vi "Rearrange Functions.vi"(11 "Functions in":T1[](array[typedef])) -> (3 "Functions in":T1[](array[typedef]))   [LabVIEW 2021, in "TAF Proj Document Type.lvlib" / "Dqmh Module.lvclass"]
uses:
  <vilib>/Wovalab/AntiDoc/Document Type/Add-ons/LabVIEW TAF Project/Dqmh Module/Dqmh Module.lvclass
  <vilib>/Wovalab/AntiDoc/Document Type/Add-ons/LabVIEW TAF Project/Dqmh Module/Requests Used By Module--cluster.ctl
  <vilib>/Wovalab/AntiDoc/Document Type/Add-ons/LabVIEW TAF Project/Project Parser/Module Fonctions--cluster.ctl
  <vilib>/Wovalab/AntiDoc/Document Type/Add-ons/LabVIEW TAF Project/Project Parser/Project Parser.lvlib
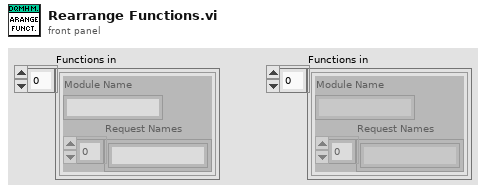
[diagram p1: front panel]
types:
  T1 = typedef "TAF Proj Document Type.lvlib/Dqmh Module.lvclass/Requests Used By Module--cluster.ctl" = cluster{"Module Name":string, "Request Names":string[]}
  T2 = typedef "TAF Proj Document Type.lvlib/Project Parser.lvlib/Module Fonctions--cluster.ctl" = cluster{"Module Name":string, "Functions":string[]}
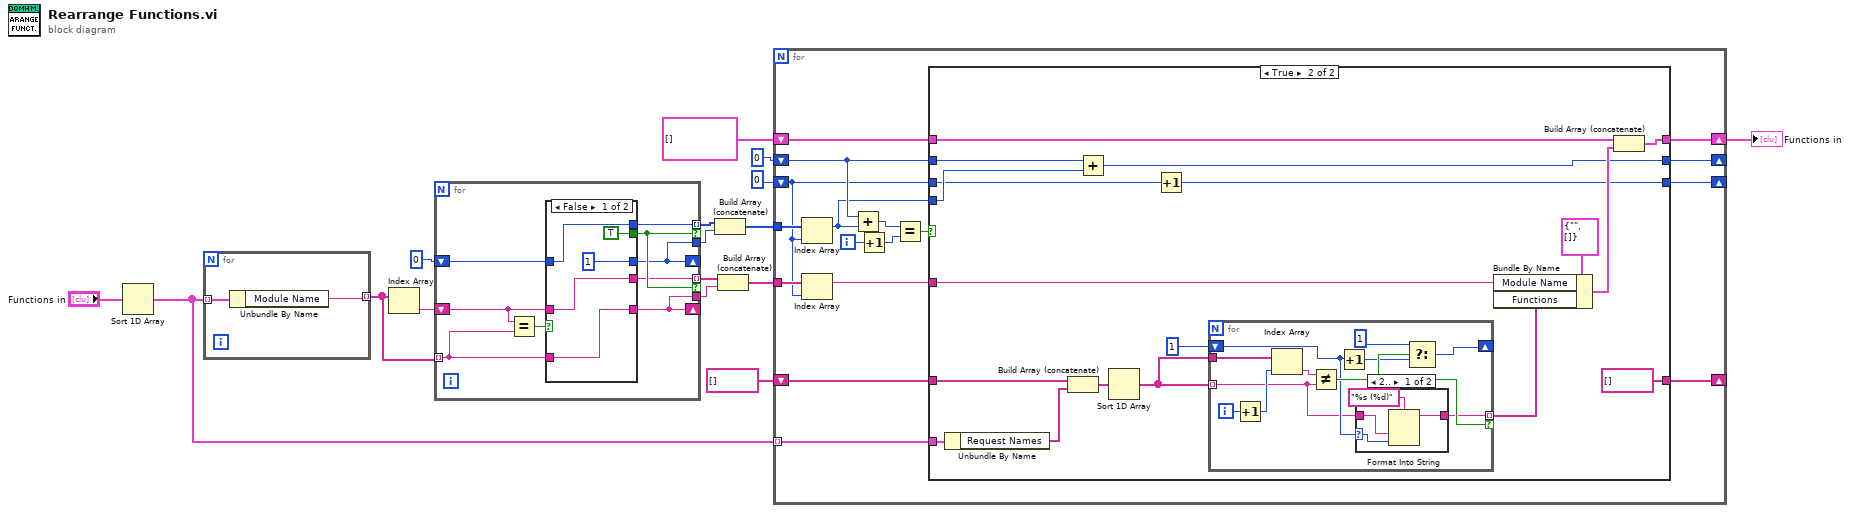
[diagram p0: block diagram]
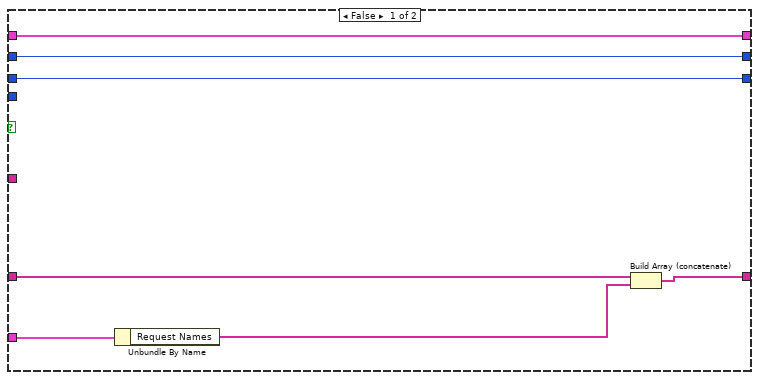
[diagram p2: hidden frame]
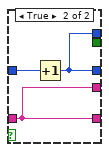
[diagram p4: hidden frame]
diagram:
  n1 = Sort 1D Array(array="Functions in") -> (sorted array=w1:T1[])
  n2 = for {
    tunnel: w1 -> [w18] mode=indexing
    tunnel: [w17] -> w11 mode=indexing
    n3 = Unbundle By Name(w18) -> ("Module Name"=w17:string)
  }
  n4 = Index Array(array=w11) -> (element=w10:string)  [unwired: 1 in]
  n5 = for {
    tunnel: w11 -> [w25] mode=indexing
    shift-right: [w19] -> _
    shift-left: w10 -> [w26]
    shift-right: [w20] -> _
    shift-left: 0 -> [w27]
    tunnel: [w22] -> w13 mode=indexing if=w24
    tunnel: [w21] -> w16 mode=indexing if=w24
    tunnel: [w20] -> w14
    tunnel: [w19] -> w15
    n6 = Equal?(x=w26, y=w25) -> (x = y?=w23:bool)
    n7 = case shown="False" w23 {
      tunnel: w27 -> [w32 w35]
      tunnel: [1 w33] -> w20
      tunnel: [w32 w33] -> w22
      tunnel: [w28 w34] -> w19
      tunnel: w25 -> [w28 _]
      tunnel: w26 -> [w29 w34]
      tunnel: [w29 w34] -> w21
      tunnel: [TRUE _] -> w24
      frame False {
      }
      frame True {
        n8 = Increment(x=w35) -> (x+1=w33:i32)
      }
    }
  }
  n9 = Build Array (concatenate)(w13, w14) -> (w6:i32[])
  n10 = Build Array (concatenate)(w16, w15) -> (w5:string[])
  n11 = for {
    tunnel: w1 -> [w36] mode=indexing
    tunnel: w5 -> [w47]
    tunnel: w6 -> [w51]
    shift-right: [w48] -> w9
    shift-left: T2[] [] ("Registred Broadcast") -> [w49]
    shift-right: [w45] -> _
    shift-left: string[] [] ("appended array") -> [w46]
    shift-right: [w43] -> _
    shift-left: 0 -> [w41]
    shift-right: [w38] -> _
    shift-left: 0 -> [w39]
    i -> [w52]
    n12 = Index Array(array=w51, index=w39) -> (element=w37:i32)
    n13 = Index Array(array=w47, index=w39) -> (element=w40:string)
    n14 = Add(x=w41, y=w37) -> (x+y=w42:i32)
    n15 = Increment(x=w52) -> (x+1=w44:i32)
    n16 = Equal?(x=w42, y=w44) -> (x = y?=w50:bool)
    n17 = case shown="True" w50 {
      tunnel: w49 -> [w59 w75]
      tunnel: [w59 w74] -> w48
      tunnel: w40 -> [_ w73]
      tunnel: w46 -> [w58 w65]
      tunnel: [w53 string[] []] -> w45
      tunnel: w37 -> [_ w72]
      tunnel: w41 -> [w57 w71]
      tunnel: [w57 w70] -> w43
      tunnel: w39 -> [w56 w69]
      tunnel: [w56 w68] -> w38
      tunnel: w36 -> [w55 w67]
      frame False {
        n18 = Unbundle By Name(w55) -> ("Request Names"=w54:string[])
        n19 = Build Array (concatenate)(w58, w54) -> (w53:string[])
      }
      frame True {
        n20 = Unbundle By Name(w67) -> ("Request Names"=w66:string[])
        n21 = Build Array (concatenate)(w65, w66) -> (w63:string[])
        n22 = Add(x=w71, y=w72) -> (x+y=w70:i32)
        n23 = Sort 1D Array(array=w63) -> (sorted array=w61:string[])
        n24 = Increment(x=w69) -> (x+1=w68:i32)
        n25 = for {
          tunnel: w61 -> [w78] mode=indexing
          tunnel: w61 -> [w88]
          tunnel: [w79] -> w60 mode=indexing if=w84
          shift-right: [w81] -> _
          shift-left: 1 -> [w80]
          i -> [w87]
          n26 = Increment(x=w87) -> (x+1=w86:i32)
          n27 = Index Array(array=w88, index=w86) -> (element=w85:string)
          n28 = Not Equal?(x=w85, y=w78) -> (x != y?=w84:bool)
          n29 = Increment(x=w80) -> (x+1=w82:i32)
          n30 = case shown="2.." w80 {
            selector: w80 -> [w90 _]
            tunnel: [w92 w93] -> w79
            tunnel: w78 -> [w91 w93]
            frame 2.. {
              n31 = Format Into String(format string="%s (%d)", w91, w90) -> (resulting string=w92:string)  [unwired: 2 in, 1 out]
            }
            frame ..1 {
            }
          }
          n32 = Select(t=1, s=w84, f=w82) -> (s? t:f=w81:i32)
        }
        n33 = Bundle By Name(cluster=T2 {"Module Name"="", "Functions"=[]} ("Module Broadcast Registred"), "Module Name"=w73, "Functions"=w60) -> (w76:T2)
        n34 = Build Array (concatenate)(w75, w76) -> (w74:T2[])
      }
    }
  }
  "Functions in" <- w9
